vi "VI Server Setup.vi"(9 "This VI":refnum<vi>, 10 "This Application":refnum<vi>, 11 "Base Event in":refnum<class "Base Event.lvclass">) -> (3 "Base Event out":refnum<class "Base Event.lvclass">)   [LabVIEW 2021, in "jettl.lvlib" / "Base Event.lvlib" / "Base Event.lvclass"]
uses:
  Base Event.lvclass
  Base Event.lvclass/Base Event.ctl
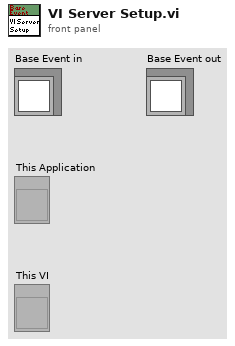
[diagram p1: front panel]
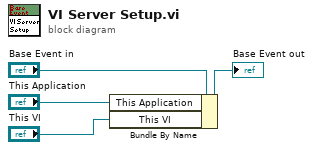
[diagram p0: block diagram]
diagram:
  n1 = Bundle By Name(cluster="Base Event in", "This Application"="This Application", "This VI"="This VI") -> (→"Base Event out":refnum<class "Base Event.lvclass">)
